vi "GET ITEM AMOUNT.vi"(11 "REFERENCES":T1) -> ()   [LabVIEW 2019]
uses:
  Controls/References Cluster.ctl
  <vilib>/userDefined/High Color/IMAQdx.ctl
  Controls/Custom Calendar/Custom Calendar.xctl
types:
  T1 = typedef "References Cluster.ctl" = cluster{"MAIN PAGES":refnum<vi>, "ADD/EDIT ITEM REFERENCES":cluster{"Identifier":refnum<vi>, "BYU ICN #":refnum<vi>, "Item Description":refnum<vi>, "Comments":refnum<vi>, "Checked Out Date":refnum<vi>, "Due Date":refnum<vi>, "Check Out Location":refnum<vi>, "Reminder Count":refnum<vi>, "Most Recent Reminder Date":refnum<vi>, "BYU ID #":refnum<vi>, "Building/Room":refnum<vi>, "Location in Room":refnum<vi>, "Manual":refnum<vi>, "Manufacturer":refnum<vi>, "Model #":refnum<vi>, "Serial #":refnum<vi>, "Date Acquired":refnum<vi>, "ADD/EDIT ITEM LABEL":refnum<vi>, "ARCHIVE ITEM":refnum<vi>, "Archive Item Inputs":refnum<vi>, "Reminder Notes":refnum<vi>, "DUPLICATE ITEM":refnum<vi>}, "ADD/EDIT USER REFERENCES":cluster{"BYU ID # (##-###-####)":refnum<vi>, "First Name":refnum<vi>, "Last Name":refnum<vi>, "Phone Number (###-###-####)":refnum<vi>, "Email":refnum<vi>, "Department":refnum<vi>, "Graduation Status":refnum<vi>, "Anticipated Graduation Year":refnum<vi>, "Credit Score":refnum<vi>, "Date Added":refnum<vi>, "Graduation Clearance Date":refnum<vi>, "Picture File Name":refnum<vi>, "ADD/EDIT USER LABEL":refnum<vi>, "Department Map":refnum<vi>, "Status Map":refnum<vi>, "Anticipated Graduation Year Map":refnum<vi>, "User Agreement":refnum<vi>, "User Comments":refnum<vi>, "Camera":refnum<vi>}, "RETURN ITEM REFERENCES":cluster{"Item or Person:":refnum<vi>, "Search Return Results":refnum<vi>, "What are you searching for?":refnum<vi>}, "SEARCH DATABASE REFERENCES":cluster{"What to Search For:":refnum<vi>, "Where to Search":refnum<vi>, "Column to Search In":refnum<vi>, "Column to Sort By":refnum<vi>, "Search Database Results":refnum<vi>, "Inventory Column Selector":refnum<vi>, "User Column Selector":refnum<vi>, "Inventory Archive Column Selector":refnum<vi>, "User Archive Column Selector":refnum<vi>, "Sales Tracking Column Selector":refnum<vi>, "Checked In Archive Column Selector":refnum<vi>, "Restore User":refnum<vi>, "Date Range":refnum<vi>, "Dates Less Than":refnum<vi>, "Dates Greater Than":refnum<vi>, "Search Print Receipt":refnum<vi>, "Edit Sale Description":refnum<vi>}, "USER ITEMS REFERENCES":cluster{"USER'S INFORMATION":refnum<vi>, "User's Checked Out Items":refnum<vi>, "User Info Comments":refnum<vi>, "SEE USER INFO COMMENTS":refnum<vi>}, "EDIT ITEMS REFERENCES":cluster{"New Check Out Location":refnum<vi>, "Items to Edit":refnum<vi>, "Edit Items Due Date":refnum<vi>, "New Reminder Notes":refnum<vi>, "New Item Description":refnum<vi>}, "CHECK OUT ITEMS REFERENCES":cluster{"Enter Item:":refnum<vi>, "Check Out Items Due Date":refnum<vi>, "Check Out Location":refnum<vi>, "Items to be Checked Out":refnum<vi>, "Possible Items":refnum<vi>, "Altered Item Description":refnum<vi>}, "TRANSFER ITEMS REFERENCES":cluster{"Search Parameter":refnum<vi>, "What to Match":refnum<vi>, "Matching Individuals":refnum<vi>, "Items to be Transferred":refnum<vi>}, "SETTINGS REFERENCES":cluster{"PSC Database Settings":refnum<vi>, "PSC Sales Item Spreadsheet":refnum<vi>}, "PSC SALES REFERENCES":cluster{"BYU ID CARD #":refnum<vi>, "Sale Description":refnum<vi>, "Scan or Enter Item Name":refnum<vi>, "Items to be Sold":refnum<vi>, "Grand Total":refnum<vi>, "Item List":refnum<vi>}}
  T2 = cluster{"BYU ID CARD #":refnum<vi>, "Sale Description":refnum<vi>, "Scan or Enter Item Name":refnum<vi>, "Items to be Sold":refnum<vi>, "Grand Total":refnum<vi>, "Item List":refnum<vi>}
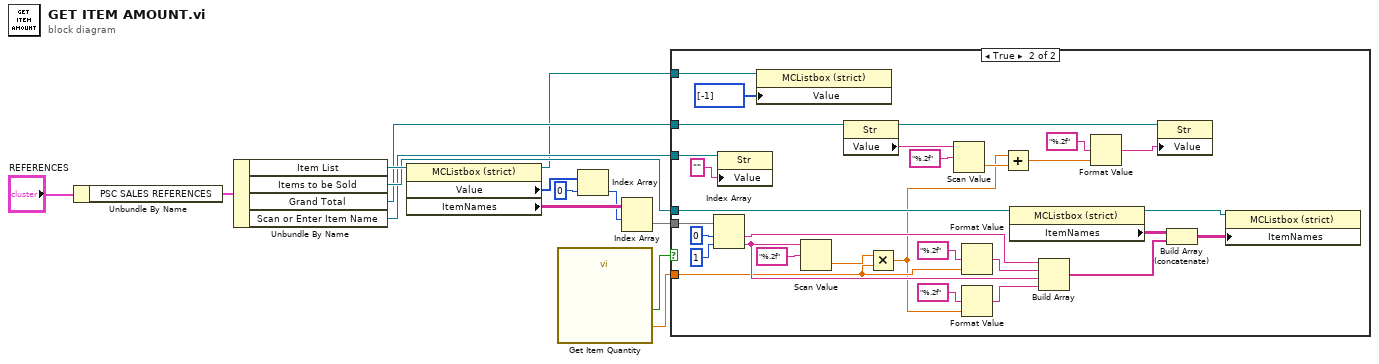
[diagram p0: block diagram]
diagram:
  n1 = Unbundle By Name("REFERENCES") -> ("PSC SALES REFERENCES"=w13:T2)
  n2 = Unbundle By Name(w13) -> ("Item List"=w12:refnum<vi>, "Items to be Sold"=w5:refnum<vi>, "Grand Total"=w4:refnum<vi>, "Scan or Enter Item Name"=w2:refnum<vi>)
  n3 = property class="MCListbox (strict)"(reference=w12) -> (reference out=w1:refnum<vi>, "Value"=w11:i32[], "ItemNames"=w9:string[][])  [unwired: 1 in, 1 out]
  n4 = call "Get Item Quantity"() -> ("Quantity"=w6:dbl, "OK"=w7:bool)  [unwired: 17 in, 1 out]
  n5 = Index Array(array=w11, index=0) -> (element=w8:i32)
  n6 = Index Array(array=w9, index (row)=w8) -> (element=w3:string[])  [unwired: 1 in]
  n7 = case shown="True" w7 {
    tunnel: w6 -> [_ w32]
    tunnel: w5 -> [_ w44]
    tunnel: w4 -> [_ w43]
    tunnel: w3 -> [_ w41]
    tunnel: w2 -> [_ w19]
    tunnel: w1 -> [_ w17]
    frame False {
    }
    frame True {
      n8 = Index Array(array=w41, index #1=0 ("index"), index #2=1 ("index")) -> (element #1=w38:string, element #2=w35:string)
      n9 = property class="Str"(reference=w19, "Value"="") -> ()  [unwired: 1 in, 2 out]
      n10 = property class="MCListbox (strict)"(reference=w17, "Value"=i32[] [-1]) -> ()  [unwired: 1 in, 2 out]
      n11 = Scan Value(string=w35, format string="%.2f") -> (value=w33:dbl)  [unwired: 1 in, 1 out]
      n12 = property class="Str"(reference=w43) -> (reference out=w26:refnum<vi>, "Value"=w30:string)  [unwired: 1 in, 1 out]
      n13 = Multiply(x=w33, y=w32) -> (x*y=w15:dbl)
      n14 = Scan Value(string=w30, format string="%.2f") -> (value=w29:dbl)  [unwired: 1 in, 1 out]
      n15 = Format Value(format string="%.2f", value (0)=w32) -> (output string=w36:string)  [unwired: 1 in]
      n16 = Format Value(format string="%.2f", value (0)=w15) -> (output string=w23:string)  [unwired: 1 in]
      n17 = Add(x=w15, y=w29) -> (x+y=w27:dbl)
      n18 = property class="MCListbox (strict)"(reference=w44) -> (reference out=w21:refnum<vi>, "ItemNames"=w42:string[][])  [unwired: 1 in, 1 out]
      n19 = Build Array(w38, w36, w35, w23) -> (w22:string[])
      n20 = Format Value(format string="%.2f", value (0)=w27) -> (output string=w25:string)  [unwired: 1 in]
      n21 = property class="Str"(reference=w26, "Value"=w25) -> ()  [unwired: 1 in, 2 out]
      n22 = Build Array (concatenate)(w42, w22) -> (w20:string[][])
      n23 = property class="MCListbox (strict)"(reference=w21, "ItemNames"=w20) -> ()  [unwired: 1 in, 2 out]
    }
  }
